vi "Defeated Message.vi"(11 "Team":refnum<class "Team.lvclass">) -> (2 "Defeated Message":string)   [LabVIEW 2020, in "SquareBattle.lvlib" / "Team.lvclass"]
doc: "Provides the message that is displayed once a team is eliminated."
uses:
  Team.lvclass
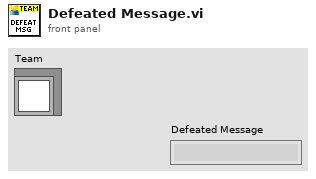
[diagram p1: front panel]
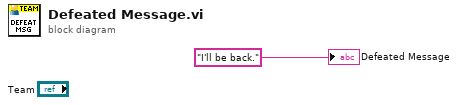
[diagram p0: block diagram]
diagram:
  "Defeated Message" <- "I'll be back." ("Victory Message")
